vi "Parameters Unit Test.vi"(8 "entrée d'erreur (pas d'erreur)":errorcluster, 9 "String":string, 10 "Label 2":string, 11 "Label":string) -> (0 "sortie d'erreur":errorcluster)   [LabVIEW 2021]
uses:
  <vilib>/addons/_JKI Toolkits/Caraya/classes/Properties.Assert/Properties.Assert.lvclass
  C:/Program Files (x86)/National Instruments/LabVIEW 2021/vi.lib/addons/_JKI Toolkits/Caraya/classes/Properties/Properties.lvclass
  <vilib>/addons/_JKI Toolkits/Caraya/classes/Assert/Assert Equal Value_Variant.vi
  <vilib>/addons/_JKI Toolkits/Caraya/classes/Assert/Assert.lvclass
  <vilib>/addons/_JKI Toolkits/Caraya/classes/Properties/Properties.lvclass
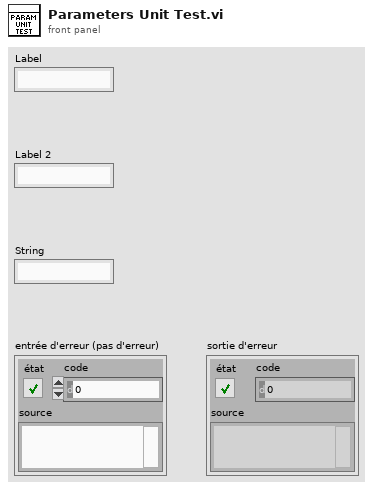
[diagram p1: front panel]
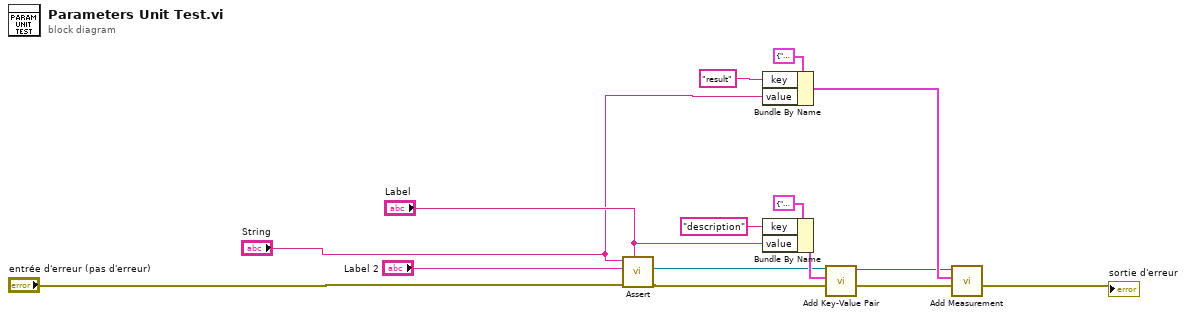
[diagram p0: block diagram]
diagram:
  n1 = call-poly <vilib>:"Assert.vi"("Label"="Label", "error in (no error)"="entrée d'erreur (pas d'erreur)", "Y"="Label 2", "X"="String") -> ("error out"=w2:errorcluster, "Properties.Assert"=w1:refnum<class "Properties.Assert.lvclass">)  [unwired: 6 in]
  n2 = Bundle By Name(cluster=cluster{"key":string, "value":variant} {"key"="", "value"=variant} ("entry"), "key"="result", "value"="String") -> (w5:cluster{"key":string, "value":variant})
  n3 = Bundle By Name(cluster=cluster{"key":string, "value":variant} {"key"="", "value"=variant} ("entry"), "key"="description", "value"="Label") -> (w8:cluster{"key":string, "value":variant})
  n4 = call <vilib>:"Add Key-Value Pair.vi"("error in (no error)"=w2, "entry"=w8, "Properties in"=w1) -> ("error out"=w4:errorcluster, "Properties out"=w3:refnum<class "Properties.Assert.lvclass">)  [unwired: 7 in]
  n5 = call <vilib>:"Add Measurement.vi"("error in (no error)"=w4, "entry"=w5, "Properties"=w3) -> ("error out"=→"sortie d'erreur":errorcluster)  [unwired: 7 in, 1 out]
